vi "FillDataTable.vi"(1 "First Data Column Index":i32, 2 "Tbl Refnum":refnum<vi>, 3 "kSAComm ref":refnum<k24>) -> ()   [LabVIEW 2019]
uses:
  C:/Users/tim/Documents/kSAComm LabView Sample/kSACommInterface.dll
  kSACommInterface.dll
panel:
  # "This VI will dynamically fill the given table based on the current marker configuration reported from the kSA acquisition app vi the GetData method.\n\nIt makes use of the internal data storage collections in the kSACommInterface assembly."
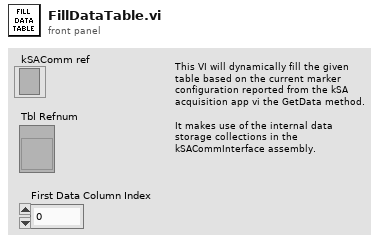
[diagram p1: front panel]
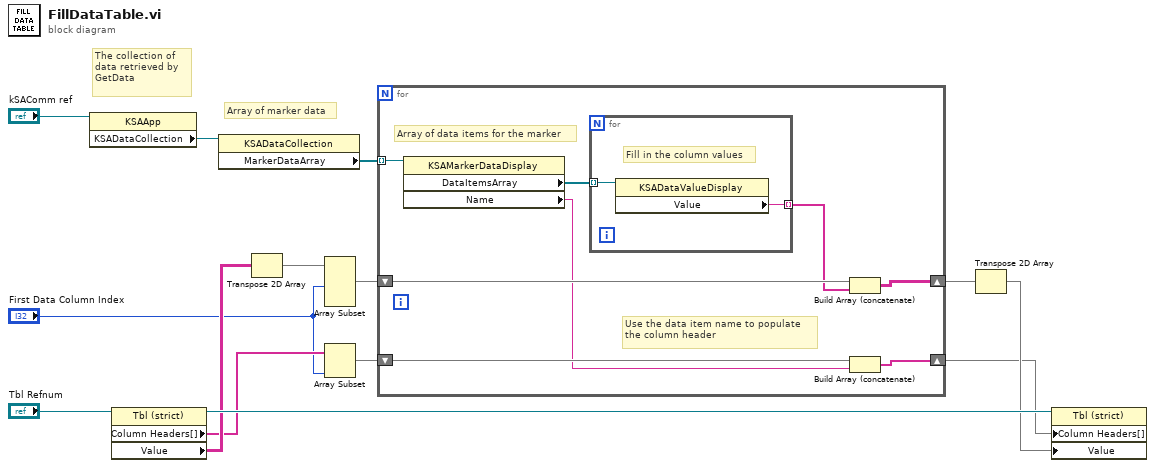
[diagram p0: block diagram]
diagram:
  # "Array of marker data"
  # "The collection of data retrieved by GetData"
  n1 = property class="KSAApp"(reference="kSAComm ref") -> ("KSADataCollection"=w13:refnum<k24>)  [unwired: 1 in, 2 out]
  n2 = property class="Tbl (strict)"(reference="Tbl Refnum") -> (reference out=w11:refnum<vi>, "Column Headers[]"=w3:string[], "Value"=w8:string[][])  [unwired: 1 in, 1 out]
  n3 = property class="KSADataCollection"(reference=w13) -> ("MarkerDataArray"=w14:refnum<k24>[])  [unwired: 1 in, 2 out]
  n4 = Transpose 2D Array(2D array=w8) -> (transposed array=w5:string[][])
  n5 = Array Subset(array=w5, length (row)="First Data Column Index") -> (w4:string[][])  [unwired: 3 in]
  n6 = Array Subset(array=w3, length="First Data Column Index") -> (w2:string[])  [unwired: 1 in]
  n7 = for {
    tunnel: w14 -> [w22] mode=indexing
    shift-right: [w17] -> w7
    shift-left: w2 -> [w16]
    shift-right: [w18] -> w9
    shift-left: w4 -> [w20]
    # "Use the data item name to populate the column header"
    # "Array of data items for the marker"
    n8 = property class="KSAMarkerDataDisplay"(reference=w22) -> ("DataItemsArray"=w21:refnum<k24>[], "Name"=w15:string)  [unwired: 1 in, 2 out]
    n9 = for {
      tunnel: w21 -> [w24] mode=indexing
      tunnel: [w23] -> w19 mode=indexing
      # "Fill in the column values"
      n10 = property class="KSADataValueDisplay"(reference=w24) -> ("Value"=w23:string)  [unwired: 1 in, 2 out]
    }
    n11 = Build Array (concatenate)(w20, w19) -> (w18:string[][])
    n12 = Build Array (concatenate)(w16, w15) -> (w17:string[])
  }
  n13 = Transpose 2D Array(2D array=w9) -> (transposed array=w10:string[][])
  n14 = property class="Tbl (strict)"(reference=w11, "Column Headers[]"=w7, "Value"=w10) -> ()  [unwired: 1 in, 2 out]
